vi "Camera-Control.vi"() -> ()   [LabVIEW 2018]
uses:
  <vilib>/userdefined/High Color/IMAQdx.ctl
  <vilib>/vision/driver/NI_Vision_Acquisition_Software.lvlib
panel:
  in  "Number of Pics":i32
  in  "String":string
  in  "File Path":path
  out "Image":T1(plugin-control)
  in  "Image Name":string="untitled"
  in  "Session In":T2
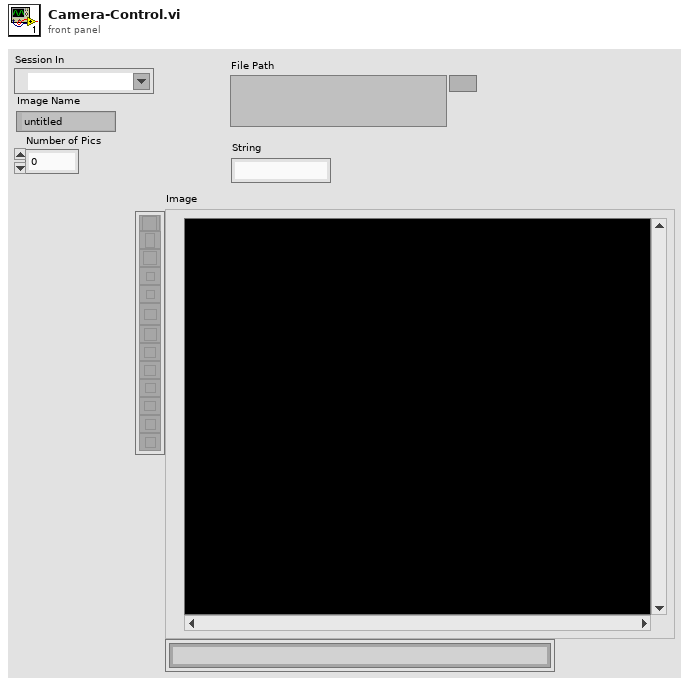
[diagram p1: front panel]
types:
  T1 = typedef "IMAQ Image.ctl" = refnum<image>
  T2 = typedef "IMAQdx.ctl" = refnum<k21>
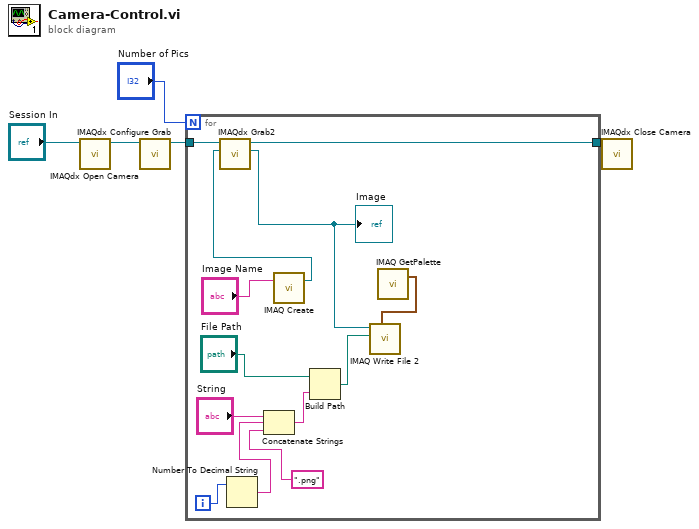
[diagram p0: block diagram]
diagram:
  n1 = call <vilib>:"IMAQdx Open Camera.vi"("Session In"="Session In") -> ("Session Out"=w3:T2)  [unwired: 9 in, 1 out]
  n2 = call <vilib>:"IMAQdx Configure Grab.vi"("Session In"=w3) -> ("Session Out"=w2:T2)  [unwired: 9 in, 1 out]
  n3 = for {
    N: "Number of Pics" -> [_]
    tunnel: w2 -> [w17]
    tunnel: [w18] -> w4
    i -> [w9]
    n4 = Number To Decimal String(number=w9) -> (decimal integer string=w8:string)  [unwired: 1 in]
    n5 = Concatenate Strings("String", w8, ".png" ("string")) -> (w10:string)
    n6 = call "IMAQ Create"("Image Name"="Image Name") -> ("New Image"=w13:T1)  [unwired: 4 in, 1 out]
    n7 = call <vilib>:"IMAQdx Grab2.vi"("Image In"=w13, "Session In"=w17) -> ("Image Out"=w15:T1, "Session Out"=w18:T2)  [unwired: 6 in, 2 out]
    "Image" <- w15
    n8 = Build Path(base path="File Path", name or relative path=w10) -> (appended path=w12:path)
    n9 = call "IMAQ GetPalette"() -> ("Color Palette"=w16:cluster{"Red":u8, "Green":u8, "Blue":u8}[])  [unwired: 5 in, 1 out]
    n10 = call-poly "IMAQ Write File 2"("Color Palette"=w16, "File Path"=w12, "Image"=w15) -> ()  [unwired: 7 in, 2 out]
  }
  n11 = call <vilib>:"IMAQdx Close Camera.vi"("Session In"=w4) -> ()  [unwired: 10 in, 1 out]
